vi "Global_CMD_CMD_Data In.vi"() -> ()   [LabVIEW 2020, in "Template_CMD.lvlib"]
uses:
  Template_CMD.lvlib
  Cluster_CMD_CMD_Data.ctl
panel:
  in  "CMD_CMD_Template_Data":T1
  # "The Names of the Data items in the Global Variable MUST describe who the Single Writer is\nFor Command Globals the Commander(CMD) represents Teleop or Autonomous or other command loop.\nThe naming convention for a Command for a Command Global is:   \n\nCMD_CMD_LibName_Data Name\n\nExample:\nCMD_CMD_BallShooter_Data\nCMD_CMD_ProgramedMotion1_Data"
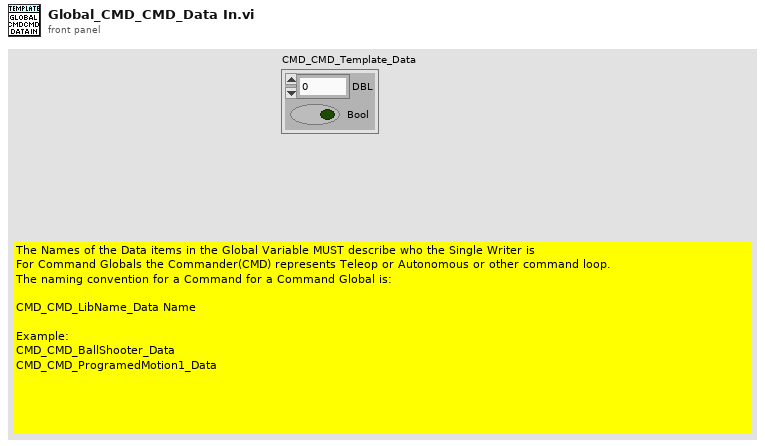
[diagram p1: front panel]
types:
  T1 = typedef "Template_CMD.lvlib/Cluster_CMD_CMD_Data.ctl" = cluster{"DBL":dbl, "Bool":bool}
diagram:
